vi "GetFilePath.vi"() -> (14 "添加的路径":path)   [LabVIEW 2019, in "User Management Model.lvclass"]
uses:
  User Management Model.lvclass
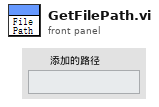
[diagram p1: front panel]
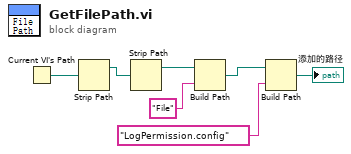
[diagram p0: block diagram]
diagram:
  n1 = Current VI's Path() -> (path=w7:path)
  n2 = Strip Path(path=w7) -> (stripped path=w3:path)  [unwired: 1 out]
  n3 = Strip Path(path=w3) -> (stripped path=w2:path)  [unwired: 1 out]
  n4 = Build Path(base path=w2, name or relative path="File" ("名称或相对路径")) -> (appended path=w5:path)
  n5 = Build Path(base path=w5, name or relative path="LogPermission.config" ("名称或相对路径")) -> (appended path=→"添加的路径":path)
